vi "Configure.vi"(8 "error in":errorcluster, 10 "name":string, 11 "PAS in":refnum<class "PAS.lvclass">) -> (0 "error out":errorcluster, 3 "PAS out":refnum<class "PAS.lvclass">)   [LabVIEW 2015, in "PAS Library.lvlib" / "PAS.lvclass"]
doc: "Configure the instrument class. If there is no config file specified, an error"
uses:
  PAS.lvclass
  Data/Main/PAS Data.lvclass
  Instrument/Instrument.lvclass/Instrument.ctl
  Data/Data.lvclass/Data.ctl
  Session APIs/File Access/Config Data/Config Data.lvclass/Config Data.ctl
  Data/Cell/PAS Cell Data.lvclass/PAS Cell Data.ctl
  PAS.lvclass/PAS.ctl
  Data/Cell/Write Ncell.vi
  Data/Write Data ID.vi
  Data/Cell/Write serializeWF_.vi
  Session APIs/File Access/Config Data/Accessors/Read Ref.vi
  Instrument/Read Data.vi
  Instrument/Read Cfg Session.vi
  Instrument/Write Data.vi
  Read Cells.vi
  Data/Main/Read CellData.vi
  Session APIs/File Access/Config Data/Read Array/Read DBL Array.vi
  <vilib>/Utility/config.llb/Read Key (I32).vi
  <vilib>/Utility/config.llb/Read Key (Boolean).vi
  Cell/Write extParams.vi
  Data/Main/Write CellData.vi
  Instrument/Instrument.lvclass
  Data/Data.lvclass
  Cell/PAS Cell.lvclass
  Session APIs/File Access/Config Data/Config Data.lvclass
  Data/Cell/PAS Cell Data.lvclass
  <vilib>/Utility/config.llb/NI_LVConfig.lvlib
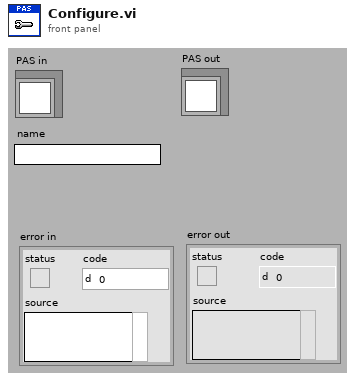
[diagram p1: front panel]
types:
  T1 = typedef "Config Data.lvclass/Config Session.ctl" = refnum<data-value>
  T2 = typedef "NI_LVConfig.lvlib/Config Data RefNum.ctl" = refnum<k1>
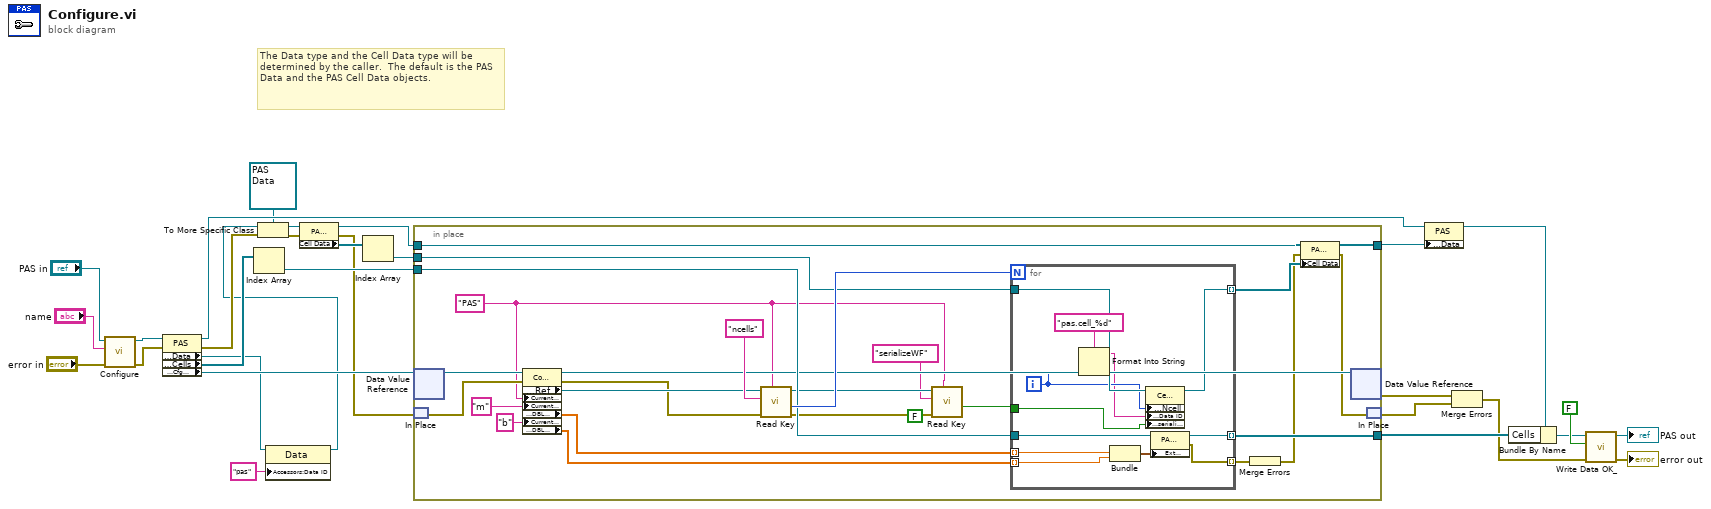
[diagram p0: block diagram]
diagram:
  # "The Data type and the Cell Data type will be determined by the caller.  The default is the PAS Data and the PAS Cell Data objects."
  n1 = call-parent "Configure.vi"("error in"="error in", "name"="name", "Instrument in"="PAS in") -> ("error out"=w26:errorcluster, "Instrument out"=w27:refnum<class "PAS.lvclass">)  [unwired: 7 in]
  n2 = property class="PAS"(reference=w27, error in=w26) -> (reference out=w16:refnum<class "PAS.lvclass">, error out=w8:errorcluster, "Accessors:Data"=w3:refnum<class "Data.lvclass">, "Data Access:Cells"=w9:refnum<class "PAS Cell.lvclass">[], "Accessors:Cfg Session"=w10:T1)
  n3 = Index Array(array=w9) -> (element=w25:refnum<class "PAS Cell.lvclass">)  [unwired: 1 in]
  n4 = property class="Data"(reference=w3, "Accessors:Data ID"="pas" ("Data ID")) -> (reference out=w2:refnum<class "Data.lvclass">)  [unwired: 1 in, 1 out]
  n5 = To More Specific Class(target class=refnum<class "PAS Data.lvclass"> refnum ("PAS Data"), reference=w2, error in=w8) -> (specific class reference=w14:refnum<class "PAS Data.lvclass">, error out=w7:errorcluster)
  n6 = property class="PAS Data"(reference=w14, error in=w7) -> (reference out=w11:refnum<class "PAS Data.lvclass">, error out=w6:errorcluster, "Cell Data"=w13:refnum<class "PAS Cell Data.lvclass">[])
  n7 = Index Array(array=w13) -> (element=w12:refnum<class "PAS Cell Data.lvclass">)  [unwired: 1 in]
  n8 = in-place {
    in-place-border: w25 -> [w53]
    in-place-border: [w52] -> w24
    in-place-border: [w48] -> w17
    in-place-border: w12 -> [w45]
    in-place-border: w11 -> [w44]
    w35 = "PAS" ("section")
    n9 = in-place-dvr #1(w10) -> (w56:refnum<class "Config Data.lvclass">)  [unwired: 1 out]
    n10 = in-place-match #2(w6) -> (w51:errorcluster)
    n11 = property class="Config Data"(reference=w56, error in=w51, "Current Section"=w35, "Current Key"="m", "Current Key"="b") -> (reference out=w39:refnum<class "Config Data.lvclass">, error out=w46:errorcluster, "Accessors:Ref"=w47:T2, "Read Array Data:DBL Data"=w41:dbl[], "Read Array Data:DBL Data"=w40:dbl[])
    n12 = call-poly <vilib>:"Read Key.vi"("section"=w35, "error in (no error)"=w46, "key"="ncells", "refnum"=w47) -> ("error out"=w33:errorcluster, "value"=w54:i32, "refnum out"=w36:T2)  [unwired: 4 in, 1 out]
    n13 = call-poly <vilib>:"Read Key.vi"("section"=w35, "error in (no error)"=w33, "default value"=FALSE, "key"="serializeWF", "refnum"=w36) -> ("value"=w32:bool)  [unwired: 3 in, 3 out]
    n14 = for {
      N: w54 -> [_]
      tunnel: w53 -> [w68]
      tunnel: [w67] -> w52 mode=indexing
      tunnel: [w66] -> w50 mode=indexing
      tunnel: [w61] -> w49 mode=indexing
      tunnel: w45 -> [w62]
      tunnel: w41 -> [w65] mode=indexing
      tunnel: w40 -> [w64] mode=indexing
      tunnel: w32 -> [w57]
      i -> [w60]
      n15 = Format Into String(format string="pas.cell_%d", w60) -> (resulting string=w58:string)  [unwired: 2 in, 1 out]
      n16 = Bundle(w65, w64) -> (w63:cluster{dbl, dbl})  [unwired: 1 in]
      n17 = property class="Cell Data"(reference=w62, "Accessors:Ncell"=w60, "Accessors:Data ID"=w58, "Accessors:serializeWF_"=w57) -> (reference out=w61:refnum<class "PAS Cell Data.lvclass">)  [unwired: 1 in, 1 out]
      n18 = property class="PAS Cell"(reference=w68, "Ext Params"=w63) -> (reference out=w67:refnum<class "PAS Cell.lvclass">, error out=w66:errorcluster)  [unwired: 1 in]
    }
    n19 = Merge Errors(w50) -> (w38:errorcluster)
    n20 = property class="PAS Data"(reference=w44, error in=w38, "Cell Data"=w49) -> (reference out=w48:refnum<class "PAS Data.lvclass">, error out=w37:errorcluster)
    n21 = in-place-dvr #1(w39) -> (w22:errorcluster)  [unwired: 1 out]
    n22 = in-place-match #2(w37) -> (w23:errorcluster)
  }
  n23 = property class="PAS"(reference=w16, "Accessors:Data"=w17) -> (reference out=w18:refnum<class "PAS.lvclass">)  [unwired: 1 in, 1 out]
  n24 = Merge Errors(w22, w23) -> (w4:errorcluster)
  n25 = Bundle By Name(cluster=w18, "Cells"=w24) -> (w19:refnum<class "PAS.lvclass">)
  n26 = call "Write Data OK_.vi"("error in (no error)"=w4, "Data OK?"=FALSE ("goodData"), "Instrument in"=w19) -> ("error out"=→"error out":errorcluster, "Instrument out"=→"PAS out":refnum<class "PAS.lvclass">)  [unwired: 7 in]
